vi "WiFi lab coordinator v1.vi"() -> ()   [LabVIEW 2016]
uses:
  VISA resource XBee.vi
panel:
  in  "Close serial comm":bool
  in  "Begin serial comm":bool
  in  "VISA resource in":refnum<visa-resource-name>
  out "Link Margin":u32
  out "Channel":u32
  out "Gateway IP":string
  out "Network Mask":string
  out "Destination IP Address":string
  out "Module IP Address":string
  out "Encryption":string
  out "SSID":string
  out "Connection Status":bool
  out "Association Information (AI)":string
  in  "Start session":bool
  in  "Protocol":enum16{"UDP", "TCP"}(ring)
  in  "Destination port (hex)":string
  in  "Source port (hex)":string
  # "Serial Port"
  # "Network Information"
  # "Session Configuration"
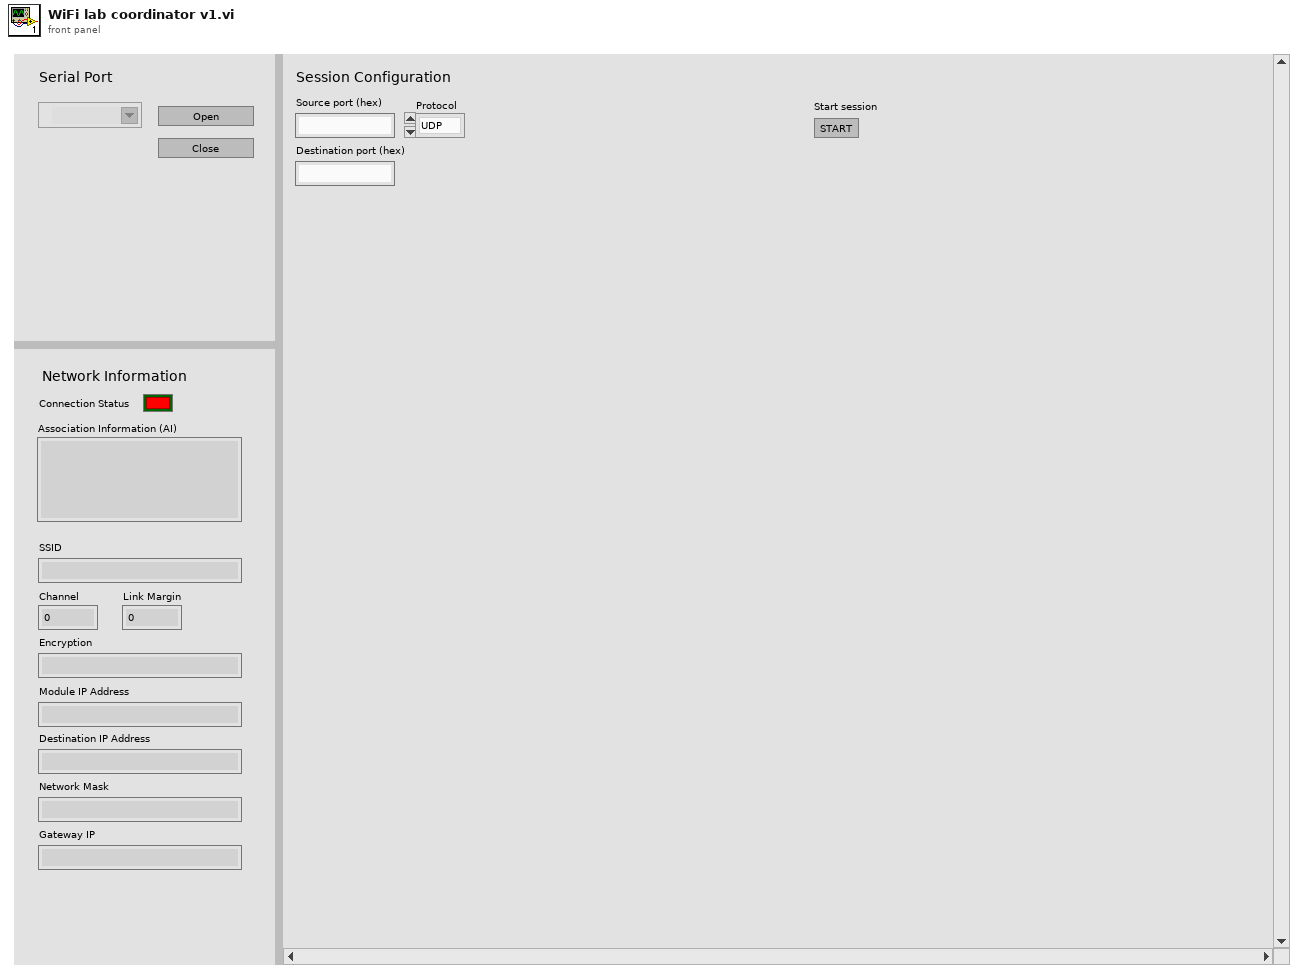
[diagram p1: front panel]
types:
  T1 = enum8{"Enabled", "Disabled", "Disabled and Grayed Out"}
  T2 = cluster{"[0]":string, "[1]":string, "[2]":string, "[3]":string, "[4]":string, "[5]":string, "[6]":string, "[7]":string, "[8]":string}
  T3 = enum32{"invalid app kind", "Development System", "Run Time System", "Student Edition", "Embedded LabVIEW", "Evaluation", "Custom"}
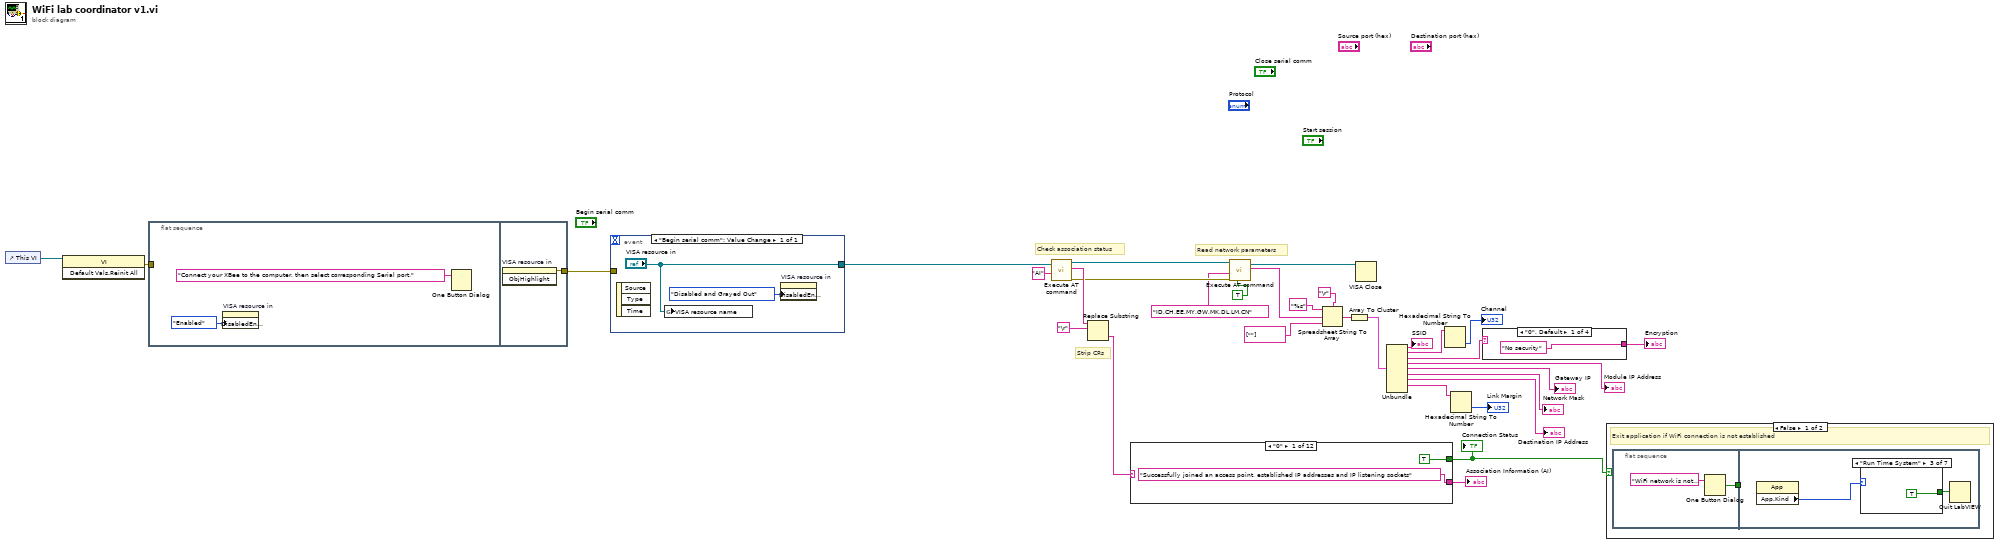
[diagram p0: block diagram]
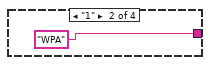
[diagram p9: hidden frame]
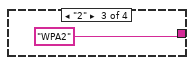
[diagram p10: hidden frame]
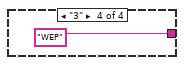
[diagram p11: hidden frame]
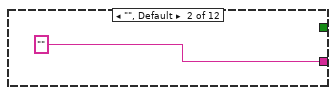
[diagram p12: hidden frame]
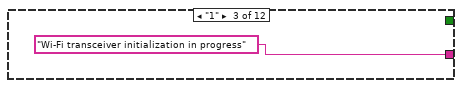
[diagram p13: hidden frame]
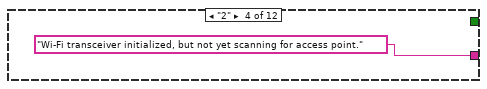
[diagram p14: hidden frame]
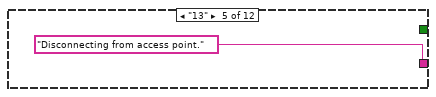
[diagram p15: hidden frame]
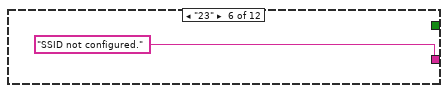
[diagram p16: hidden frame]
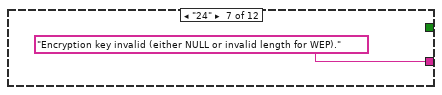
[diagram p17: hidden frame]
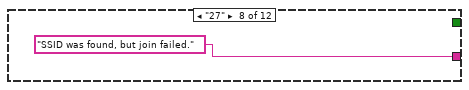
[diagram p18: hidden frame]
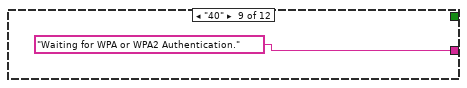
[diagram p19: hidden frame]
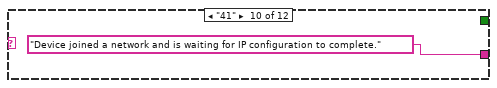
[diagram p20: hidden frame]
diagram:
  # "Read network parameters"
  # "Strip CRs"
  # "Check association status"
  n1 = control-ref of="This VI"() -> (w4:refnum<vi>)
  n2 = invoke class="VI" method="Default Vals.Reinit All"(reference=w4) -> (error out=w3:errorcluster)  [unwired: 2 in, 2 out]
  n3 = flat-sequence {
    tunnel: w3 -> [_]
    tunnel: [w35] -> w1
    frame #0 {
      n4 = property on="VISA resource in" class="VISAName"("DisabledEnum"=T1."Enabled" ("Disabled")) -> ()  [unwired: 2 in, 2 out]
      n5 = One Button Dialog(message="Connect your XBee to the computer, then select corresponding Serial port.") -> ()  [unwired: 1 in, 1 out]
    }
    frame #1 {
      n6 = invoke on="VISA resource in" class="VISAName" method="ObjHighlight"() -> (error out=w35:errorcluster)  [unwired: 3 in, 2 out]
    }
  }
  n7 = event shown="[0] \"Begin serial comm\": Value Change" {
    selector: _ -> [_]
    dyn-events: _ -> [_]
    timeout: _ -> [_]
    tunnel: ["VISA resource in"] -> w2
    tunnel: w1 -> [_]
    event "Begin serial comm": Value Change {
      n8 = event-data() -> ()  [unwired: 1 in, 3 out]
      n9 = global write "VISA resource XBee.vi" "VISA resource name"("VISA resource in") -> ()
      n10 = property on="VISA resource in" class="VISAName"("DisabledEnum"=T1."Disabled and Grayed Out" ("Disabled")) -> ()  [unwired: 2 in, 2 out]
    }
  }
  n11 = call "Execute AT command.vi"("AT Command"="AI", "VISA resource in"=w2) -> ("error out"=w26:errorcluster, "Response message"=w31:string, "VISA resource out"=w27:refnum<visa-resource-name>)  [unwired: 6 in]
  n12 = Replace Substring(4:"\r", 5:w31) -> (0:w28:string)  [unwired: 2 in, 1 out]
  n13 = case shown="\"0\"" w28 {
    tunnel: ["Successfully joined an access point, established IP addresses and IP listening sockets" "" "Wi-Fi transceiver initialization in progress" "Wi-Fi transceiver initialized, but not yet scanning for access point." "Disconnecting from access point." "SSID not configured." "Encryption key invalid (either NULL or invalid length for WEP)." "SSID was found, but join failed." "Waiting for WPA or WPA2 Authentication." "Device joined a network and is waiting for IP configuration to complete." "Device is joined, IP is configured, and listening sockets are being set up" "Device is currently scanning for the configured SSID."] -> w29
    tunnel: [TRUE _ _ _ _ _ _ _ _ _ _ _] -> w5
    frame "0" {
    }
    frame "", Default {
    }
    frame "1" {
    }
    frame "2" {
    }
    frame "13" {
    }
    frame "23" {
    }
    frame "24" {
    }
    frame "27" {
    }
    frame "40" {
    }
    frame "41" {
    }
    frame "42" {
    }
    frame "FF" {
    }
  }
  "Association Information (AI)" <- w29
  "Connection Status" <- w5
  n14 = call "Execute AT command.vi"("Exit AT mode"=TRUE, "error in (no error)"=w26, "AT Command"="ID,CH,EE,MY,GW,MK,DL,LM,CN", "VISA resource in"=w27) -> ("Response message"=w23:string, "VISA resource out"=w6:refnum<visa-resource-name>)  [unwired: 4 in, 1 out]
  n15 = Spreadsheet String To Array(delimiter (Tab)="\r", format string="%s", spreadsheet string=w23, array type (2D Dbl)=string[] [""]) -> (array=w19:string[])
  n16 = Array To Cluster(array=w19) -> (cluster=w18:T2)
  n17 = VISA Close(VISA resource name=w6) -> ()  [unwired: 1 in, 1 out]
  n18 = Unbundle(w18) -> ("[0]"=→"SSID":string, "[1]"=w12:string, "[2]"=w8:string, "[3]"=→"Module IP Address":string, "[4]"=→"Gateway IP":string, "[5]"=→"Network Mask":string, "[6]"=→"Destination IP Address":string, "[7]"=w9:string)  [unwired: 1 out]
  n19 = Hexadecimal String To Number(string=w12) -> (number=→"Channel":u32)  [unwired: 2 in, 1 out]
  n20 = Hexadecimal String To Number(string=w9) -> (number=→"Link Margin":u32)  [unwired: 2 in, 1 out]
  n21 = case shown="\"0\", Default" w8 {
    tunnel: ["No security" ("format string") "WPA" "WPA2" "WEP"] -> w7
    frame "0", Default {
    }
    frame "1" {
    }
    frame "2" {
    }
    frame "3" {
    }
  }
  "Encryption" <- w7
  n22 = case shown="False" w5 {
    frame False {
      # "Exit application if WiFi connection is not established"
      n23 = flat-sequence {
        tunnel: [w56] -> w55
        tunnel: w55 -> [_]
        frame #0 {
          n24 = One Button Dialog(message="WiFi network is not configured. Please use XCTU to connect to WiFI network first. The application will close.") -> (true=w56:bool)  [unwired: 1 in]
        }
        frame #1 {
          n25 = property class="App"() -> ("App.Kind"=w59:T3)  [unwired: 2 in, 2 out]
          n26 = case shown="\"Run Time System\"" w59 {
            tunnel: [_ _ TRUE _ _ _ _] -> w58
            frame "invalid app kind", Default {
            }
            frame "Development System" {
            }
            frame "Run Time System" {
            }
            frame "Student Edition" {
            }
            frame "Embedded LabVIEW" {
            }
            frame "Evaluation" {
            }
            frame "Custom" {
            }
          }
          n27 = Quit LabVIEW(quit? (T)=w58) -> ()
        }
      }
    }
    frame True {
      # "Do nothing if WiFi connection is established"
    }
  }
